vi "Convert Absolute Move to String.vi"(9 "Y":i32, 11 "X":i32) -> (3 "String":string)   [LabVIEW 2020, in "MacroAssert.lvlib" / "Mouse Action.lvclass"]
uses:
  Mouse Action.lvclass
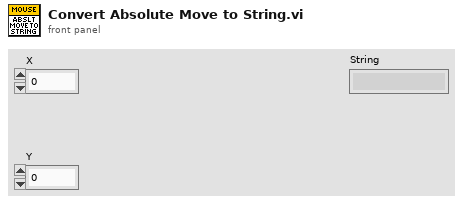
[diagram p1: front panel]
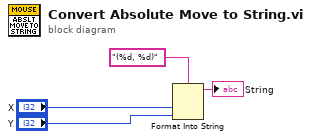
[diagram p0: block diagram]
diagram:
  n1 = Format Into String(format string="(%d, %d)", "X", "Y") -> (resulting string=→"String":string)  [unwired: 2 in, 1 out]
